vi "Load ROM.vi"(8 "error in (no error)":errorcluster, 10 "ROM":path, 11 "EEPROM in":refnum<class "EEPROM.lvclass">) -> (0 "error out":errorcluster, 3 "EEPROM out":refnum<class "EEPROM.lvclass">)   [LabVIEW 2021, in "EEPROM.lvclass"]
uses:
  EEPROM.lvclass
  EEPROM.lvclass/EEPROM.ctl
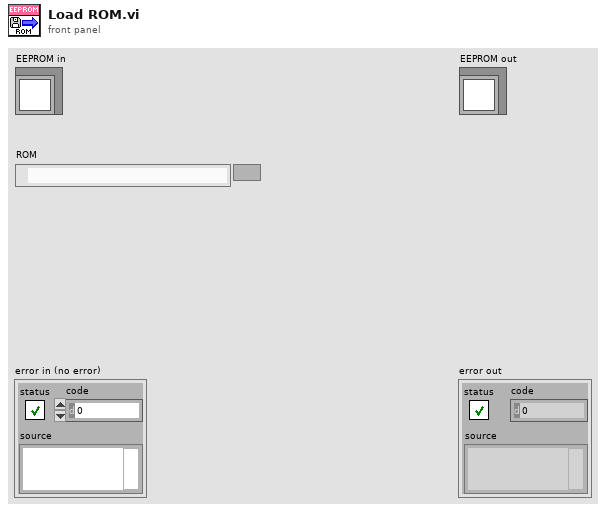
[diagram p1: front panel]
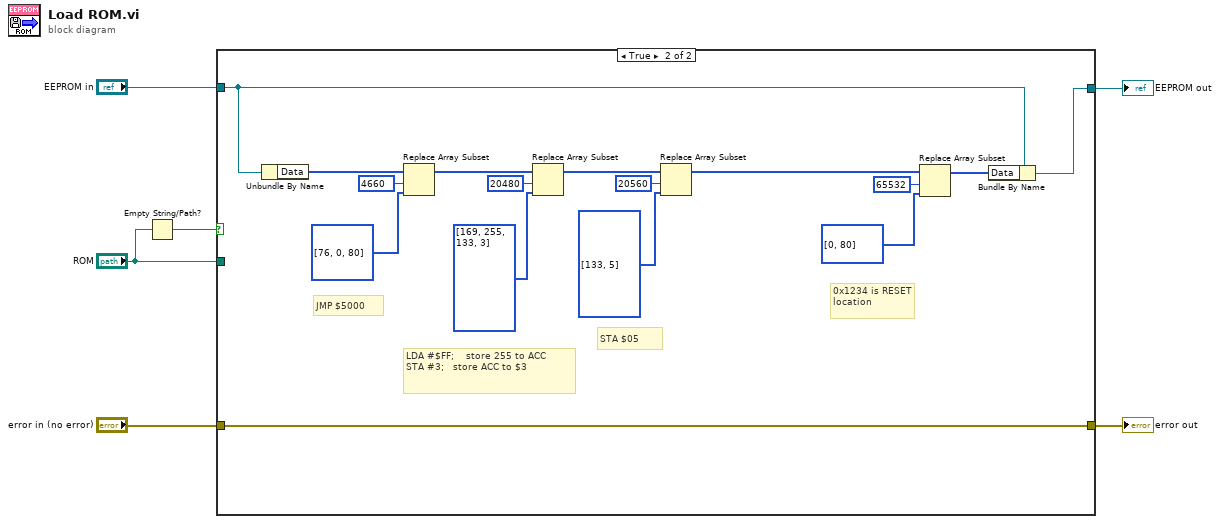
[diagram p0: block diagram]
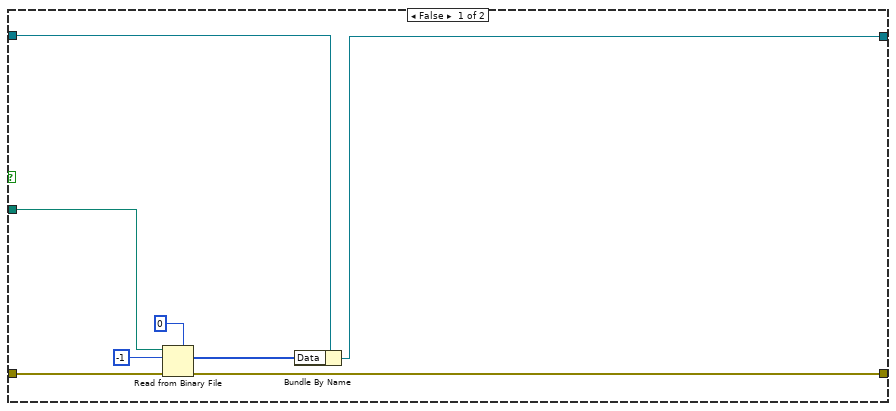
[diagram p2: hidden frame]
diagram:
  n1 = Empty String/Path?(string/path="ROM") -> (empty?=w4:bool)
  n2 = case shown="True" w4 {
    tunnel: "EEPROM in" -> [w10 w18]
    tunnel: [w9 w16] -> w5
    tunnel: "error in (no error)" -> [w14 w15]
    tunnel: "ROM" -> [w13 _]
    tunnel: [w8 w15] -> w1
    frame False {
      n3 = Read from Binary File(5:u8 0, 8:w14, 10:-1 ("count (1)"), 11:w13) -> (0:w8:errorcluster, 2:w7:u8[])  [unwired: 2 in, 2 out]
      n4 = Bundle By Name(cluster=w10, "Data"=w7) -> (w9:refnum<class "EEPROM.lvclass">)
    }
    frame True {
      # "STA $05"
      # "LDA #$FF;    store 255 to ACC\nSTA #3;   store ACC to $3"
      # "0x1234 is RESET location"
      # "JMP $5000"
      n5 = Unbundle By Name(w18) -> ("Data"=w19:u8[])
      n6 = Replace Array Subset(array=w19, new element=u8[] [76, 0, 80], index=u16 4660) -> (w24:u8[])
      n7 = Replace Array Subset(array=w24, new element=u8[] [169, 255, 133, 3], index=20480) -> (w28:u8[])
      n8 = Replace Array Subset(array=w28, new element=u8[] [133, 5], index=20560) -> (w30:u8[])
      n9 = Replace Array Subset(array=w30, new element=u8[] [0, 80], index=u16 65532) -> (w17:u8[])
      n10 = Bundle By Name(cluster=w18, "Data"=w17) -> (w16:refnum<class "EEPROM.lvclass">)
    }
  }
  "error out" <- w1
  "EEPROM out" <- w5
